vi "Browsing整体图.vi"() -> ()   [LabVIEW 2014]
panel:
  in  "Mozilla":bool
  in  "Lock":bool
  in  "Local network":bool
  in  "Irc":bool
  in  "Important":bool
  in  "Icq":bool
  in  "Home":bool
  in  "Get":bool
  in  "Game":bool
  in  "Ftp":bool
  in  "Folder":bool
  in  "Firebird":bool
  in  "Exec":bool
  in  "Download":bool
  in  "Device":bool
  in  "Cookie":bool
  in  "Contact":bool
  in  "Chat":bool
  in  "Browsing":bool
  in  "Browser":bool
  in  "Address":bool
  in  "Add":bool
  in  "Www":bool
  in  "World":bool
  in  "Thunderbird":bool
  in  "Socket":bool
  in  "Services":bool
  in  "Server":bool
  in  "Remove":bool
  in  "Opera":bool
  in  "Network":bool
  in  "Netscape":bool
  in  "My network":bool
  in  "My computer":bool
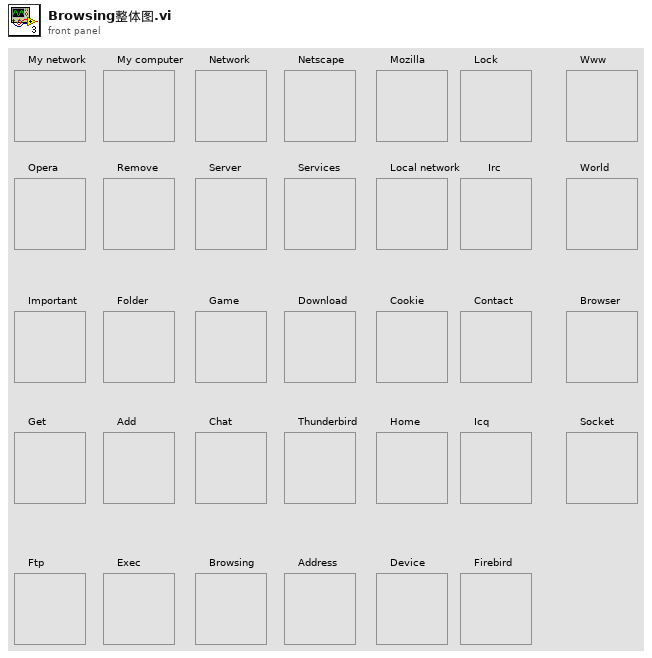
[diagram p1: front panel]
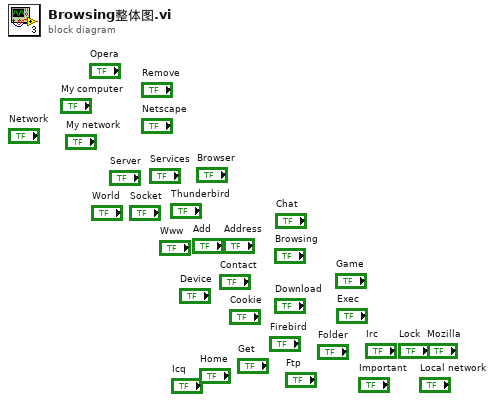
[diagram p0: block diagram]
diagram:
